vi "Teleop - shooter (SubVI).vi"(0 "Shoot":bool, 1 "inAuto":bool, 2 "AutoTurret":dbl, 7 "Desired cluster In":T1 {"shooterMotorMode" items=["PercentOutput"=0, "Position"=1, "Velocity"=2, "Current"=3, "Follower"=5, "MotionProfile"=6, "MotionMagic"=7, "MotionProfileArc"=10, "Disabled"=15]}, 9 "Constant Cluster":T4 {"12. Auton Deriv Drive Straight Gain" format="%_6f"; "11. Auton Int Drive Straight Gain" format="%_6f"; "10. Auton Prop Drive Straight Gain" format="%_6f"; "9. Auton I Output Limit Turn Gain" format="%_6f"; "8. Auton Deriv Turn Gain" format="%_6f"; "7. Auton Int Turn Gain" format="%_6f"; "1. Auton Prop Drive Gain" format="%_6f"; "2. Auton Int Drive Gain" format="%_6f"; "3. Auton Deriv Drive Gain" format="%_6f"; "4. I Output Drive  Limit" format="%_6f"; "5. Auto Drive Cheat (%)" format="%_6f"; "6. Auton Prop Turn Gain" format="%_6f"}, 11 "Sensors In":T5, 12 "wallShoot":bool, 14 "wallShootDistanceReached":bool) -> (4 "Shooting Conditions":T3, 8 "Desired cluster out":T1 {"shooterMotorMode" items=["PercentOutput"=0, "Position"=1, "Velocity"=2, "Current"=3, "Follower"=5, "MotionProfile"=6, "MotionMagic"=7, "MotionProfileArc"=10, "Disabled"=15]}, 10 "Constant Cluster Out":T4 {"12. Auton Deriv Drive Straight Gain" format="%_6f"; "11. Auton Int Drive Straight Gain" format="%_6f"; "10. Auton Prop Drive Straight Gain" format="%_6f"; "9. Auton I Output Limit Turn Gain" format="%_6f"; "8. Auton Deriv Turn Gain" format="%_6f"; "7. Auton Int Turn Gain" format="%_6f"; "1. Auton Prop Drive Gain" format="%_6f"; "2. Auton Int Drive Gain" format="%_6f"; "3. Auton Deriv Drive Gain" format="%_6f"; "4. I Output Drive  Limit" format="%_6f"; "5. Auto Drive Cheat (%)" format="%_6f"; "6. Auton Prop Turn Gain" format="%_6f"}, 15 "Sensors Out":T5)   [LabVIEW 2019]
uses:
  Autonomous/TypeDefs/Sensor TypeDef.ctl
  Disabled/Constant VI_s/Disabled - Constant Cluster Typedef.ctl
  Desired Cluster.ctl
  <vilib>/Rock Robotics/WPI/ThirdParty/Phoenix-LabVIEW/Motor Controller/Controls/CTRE_Phoenix_MotorControl_ControlMode.ctl
  <vilib>/Rock Robotics/Network Tables/NT Write Number.vi
panel:
  in  "input cluster":T3
  out "Wall Shot Shooter\nSpeed in Range":bool
  out "Wall Shot Turrent\nAngle in Range":bool
  out "Wall Shot Hood\nAngle in Range":bool
  out "Shooter Speed\nin Shooting Range":bool
  out "Turret Angle In\nShooting Range":bool
  out "Hood Angle In\nShooting Range":bool
  out "v*slope multiple":dbl
  out "x*slope multiple":dbl
  in  "v slope":dbl=0.35
  in  "x slope":dbl=-1.5
  out "desired hood angle":dbl
  out "velocity":dbl
  out "Horizontal Distance\nTo Target":dbl
  # "Inputs"
  # "Outputs"
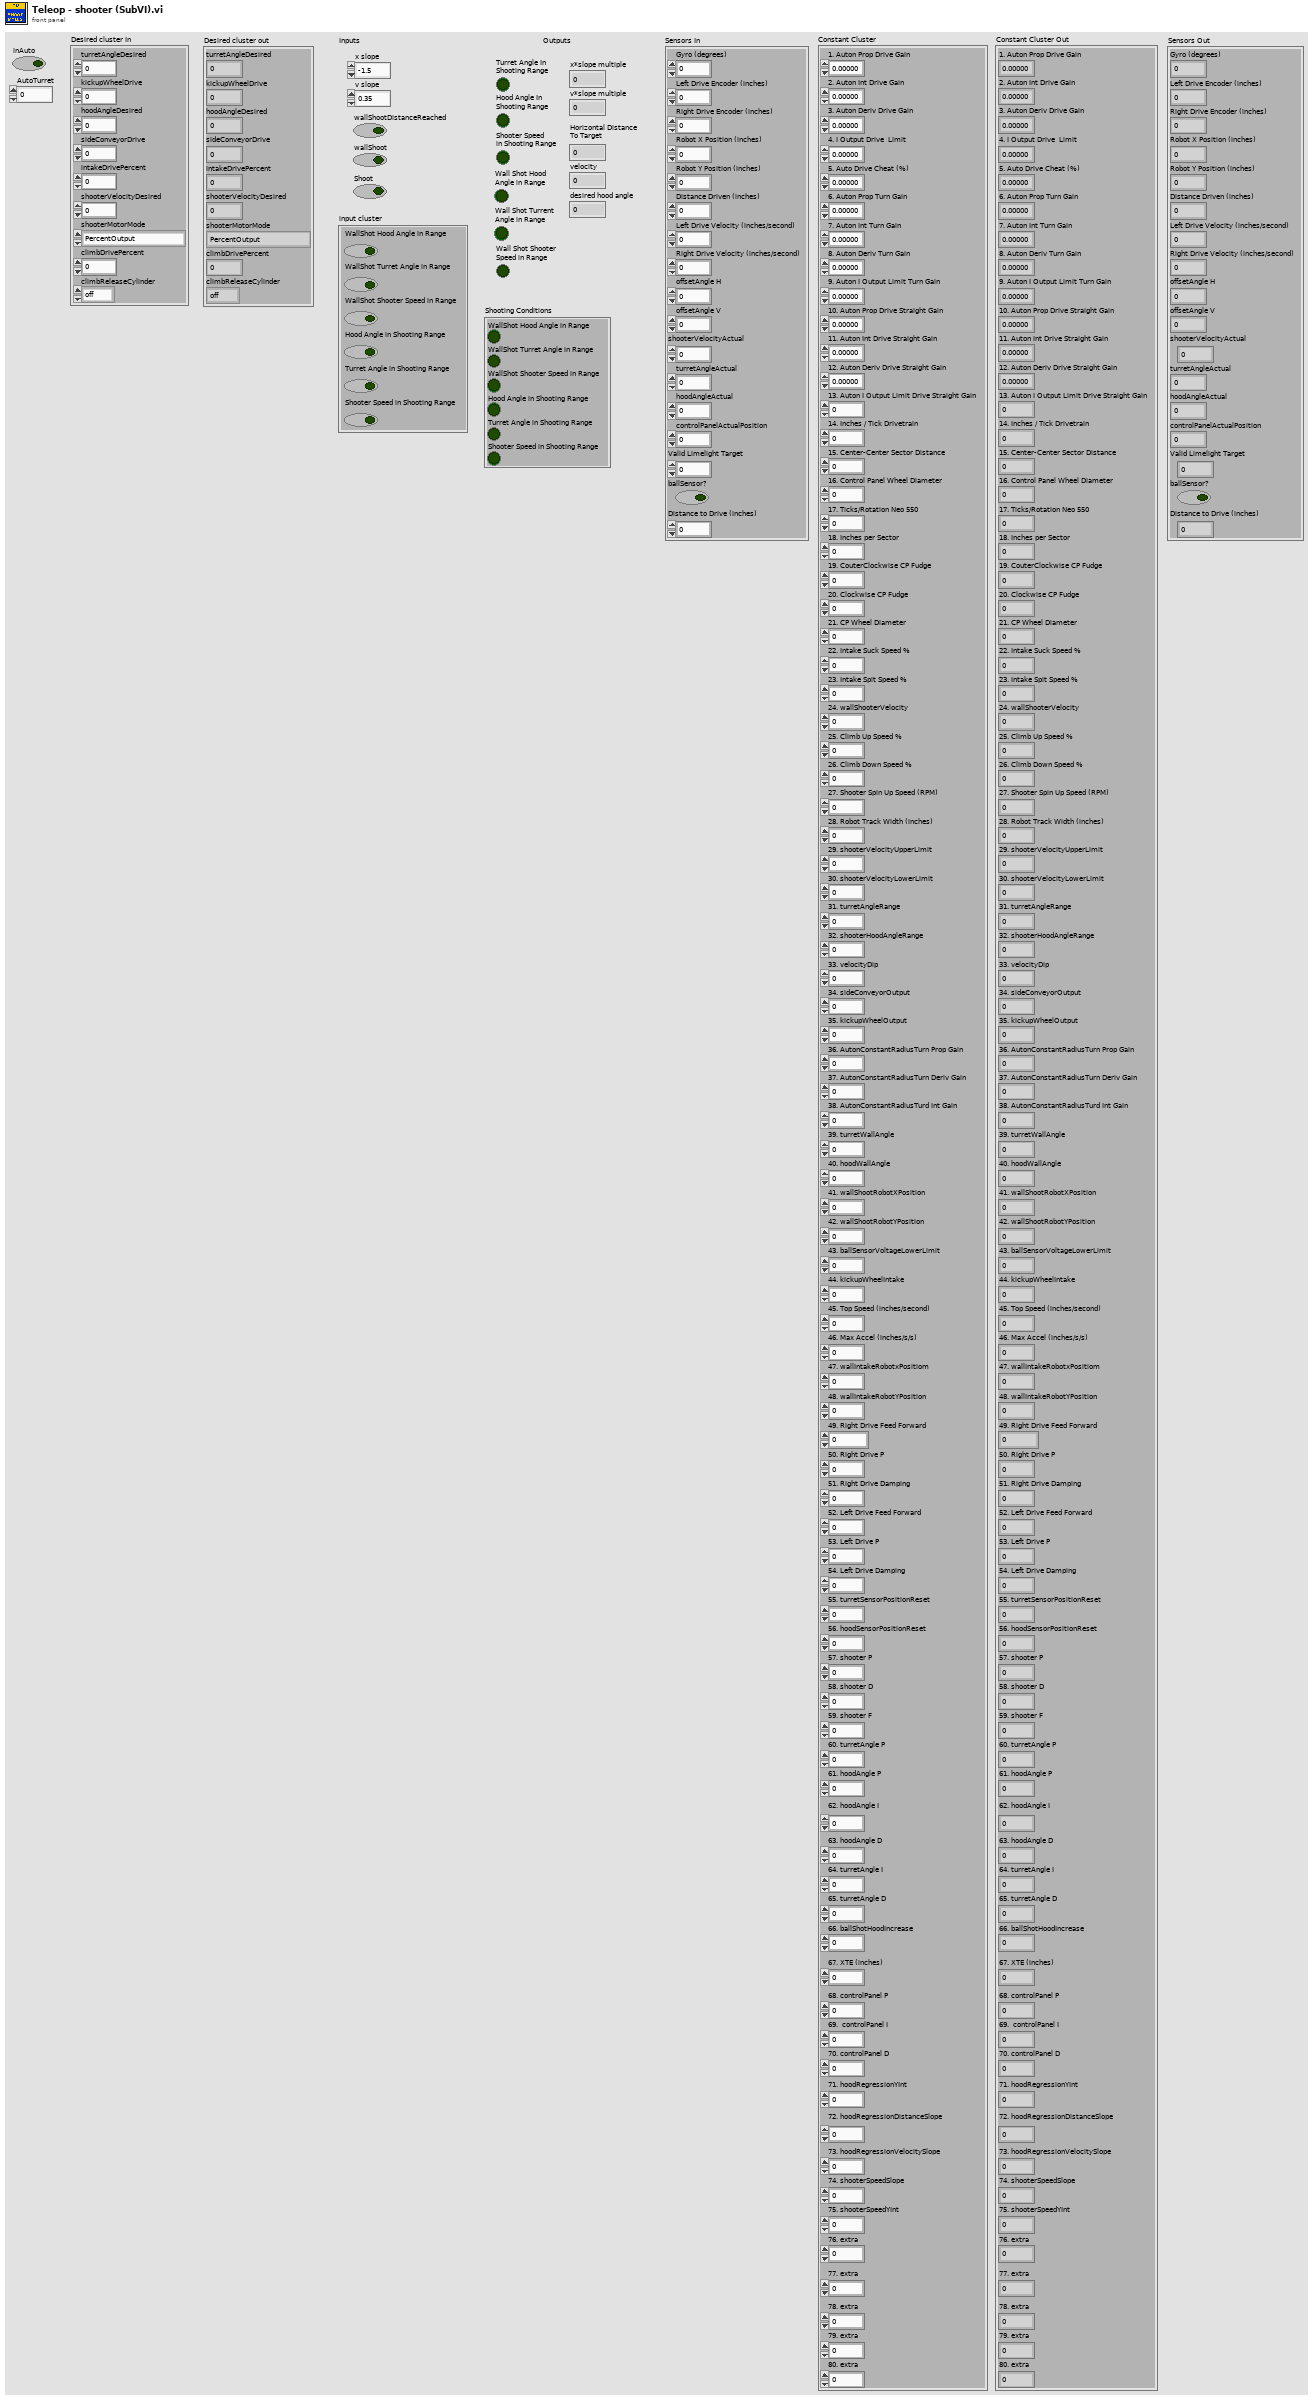
[diagram p1: front panel]
types:
  T1 = typedef "Desired Cluster.ctl" = cluster{"turretAngleDesired":dbl, "kickupWheelDrive":dbl, "hoodAngleDesired":dbl, "sideConveyorDrive":dbl, "intakeDrivePercent":dbl, "shooterVelocityDesired":dbl, "shooterMotorMode":T2, "climbDrivePercent":dbl, "climbReleaseCylinder":enum16{"off", "on", "forward", "back"}}
  T2 = typedef "CTRE_Phoenix_MotorControl_ControlMode.ctl" = u16
  T3 = cluster{"WallShot Hood Angle in Range":bool, "WallShot Turret Angle in Range":bool, "WallShot Shooter Speed in Range":bool, "Hood Angle in Shooting Range":bool, "Turret Angle in Shooting Range":bool, "Shooter Speed in Shooting Range":bool}
  T4 = typedef "Disabled - Constant Cluster Typedef.ctl" = cluster{"1. Auton Prop Drive Gain":dbl, "2. Auton Int Drive Gain":dbl, "3. Auton Deriv Drive Gain":dbl, "4. I Output Drive  Limit":dbl, "5. Auto Drive Cheat (%)":dbl, "6. Auton Prop Turn Gain":dbl, "7. Auton Int Turn Gain":dbl, "8. Auton Deriv Turn Gain":dbl, "9. Auton I Output Limit Turn Gain":dbl, "10. Auton Prop Drive Straight Gain":dbl, "11. Auton Int Drive Straight Gain":dbl, "12. Auton Deriv Drive Straight Gain":dbl, "13. Auton I Output Limit Drive Straight Gain":dbl, "14. Inches / Tick Drivetrain":dbl, "15. Center-Center Sector Distance":dbl, "16. Control Panel Wheel Diameter":dbl, "17. Ticks/Rotation Neo 550":dbl, "18. Inches per Sector":dbl, "19. CouterClockwise CP Fudge":dbl, "20. Clockwise CP Fudge":dbl, "21. CP Wheel Diameter":dbl, "22. Intake Suck Speed %":dbl, "23. Intake Spit Speed %":dbl, "24. wallShooterVelocity":dbl, "25. Climb Up Speed %":dbl, "26. Climb Down Speed %":dbl, "27. Shooter Spin Up Speed (RPM)":dbl, "28. Robot Track Width (inches)":dbl, "29. shooterVelocityUpperLimit":dbl, "30. shooterVelocityLowerLimit":dbl, "31. turretAngleRange":dbl, "32. shooterHoodAngleRange":dbl, "33. velocityDip":dbl, "34. sideConveyorOutput":dbl, "35. kickupWheelOutput":dbl, "36. AutonConstantRadiusTurn Prop Gain":dbl, "37. AutonConstantRadiusTurn Deriv Gain":dbl, "38. AutonConstantRadiusTurd Int Gain":dbl, "39. turretWallAngle":dbl, "40. hoodWallAngle":dbl, "41. wallShootRobotXPosition":dbl, "42. wallShootRobotYPosition":dbl, "43. ballSensorVoltageLowerLimit":dbl, "44. kickupWheelIntake":dbl, "45. Top Speed (inches/second)":dbl, "46. Max Accel (inches/s/s)":dbl, "47. wallIntakeRobotxPositiom":dbl, "48. wallIntakeRobotYPosition":dbl, "49. Right Drive Feed Forward":dbl, "50. Right Drive P":dbl, "51. Right Drive Damping":dbl, "52. Left Drive Feed Forward":dbl, "53. Left Drive P":dbl, "54. Left Drive Damping":dbl, "55. turretSensorPositionReset":dbl, "56. hoodSensorPositionReset":dbl, "57. shooter P":dbl, "58. shooter D":dbl, "59. shooter F":dbl, "60. turretAngle P":dbl, "61. hoodAngle P":dbl, "62. hoodAngle I":dbl, "63. hoodAngle D":dbl, "64. turretAngle I":dbl, "65. turretAngle D":dbl, "66. ballShotHoodIncrease":dbl, "67. XTE (inches)":dbl, "68. controlPanel P":dbl, "69.  controlPanel I":dbl, "70. controlPanel D":dbl, "71. hoodRegressionYInt":dbl, "72. hoodRegressionDistanceSlope":dbl, "73. hoodRegressionVelocitySlope":dbl, "74. shooterSpeedSlope":dbl, "75. shooterSpeedYInt":dbl, "76. extra":dbl, "77. extra":dbl, "78. extra":dbl, "79. extra":dbl, "80. extra":dbl}
  T5 = typedef "Sensor TypeDef.ctl" = cluster{"Gyro (degrees)":dbl, "Left Drive Encoder (inches)":dbl, "Right Drive Encoder (inches)":dbl, "Robot X Position (inches)":dbl, "Robot Y Position (inches)":dbl, "Distance Driven (inches)":dbl, "Left Drive Velocity (inches/second)":dbl, "Right Drive Velocity (inches/second)":dbl, "offsetAngle H":dbl, "offsetAngle V":dbl, "shooterVelocityActual":dbl, "turretAngleActual":dbl, "hoodAngleActual":dbl, "controlPanelActualPosition":dbl, "Valid Limelight Target":dbl, "ballSensor?":bool, "Distance to Drive (inches)":dbl}
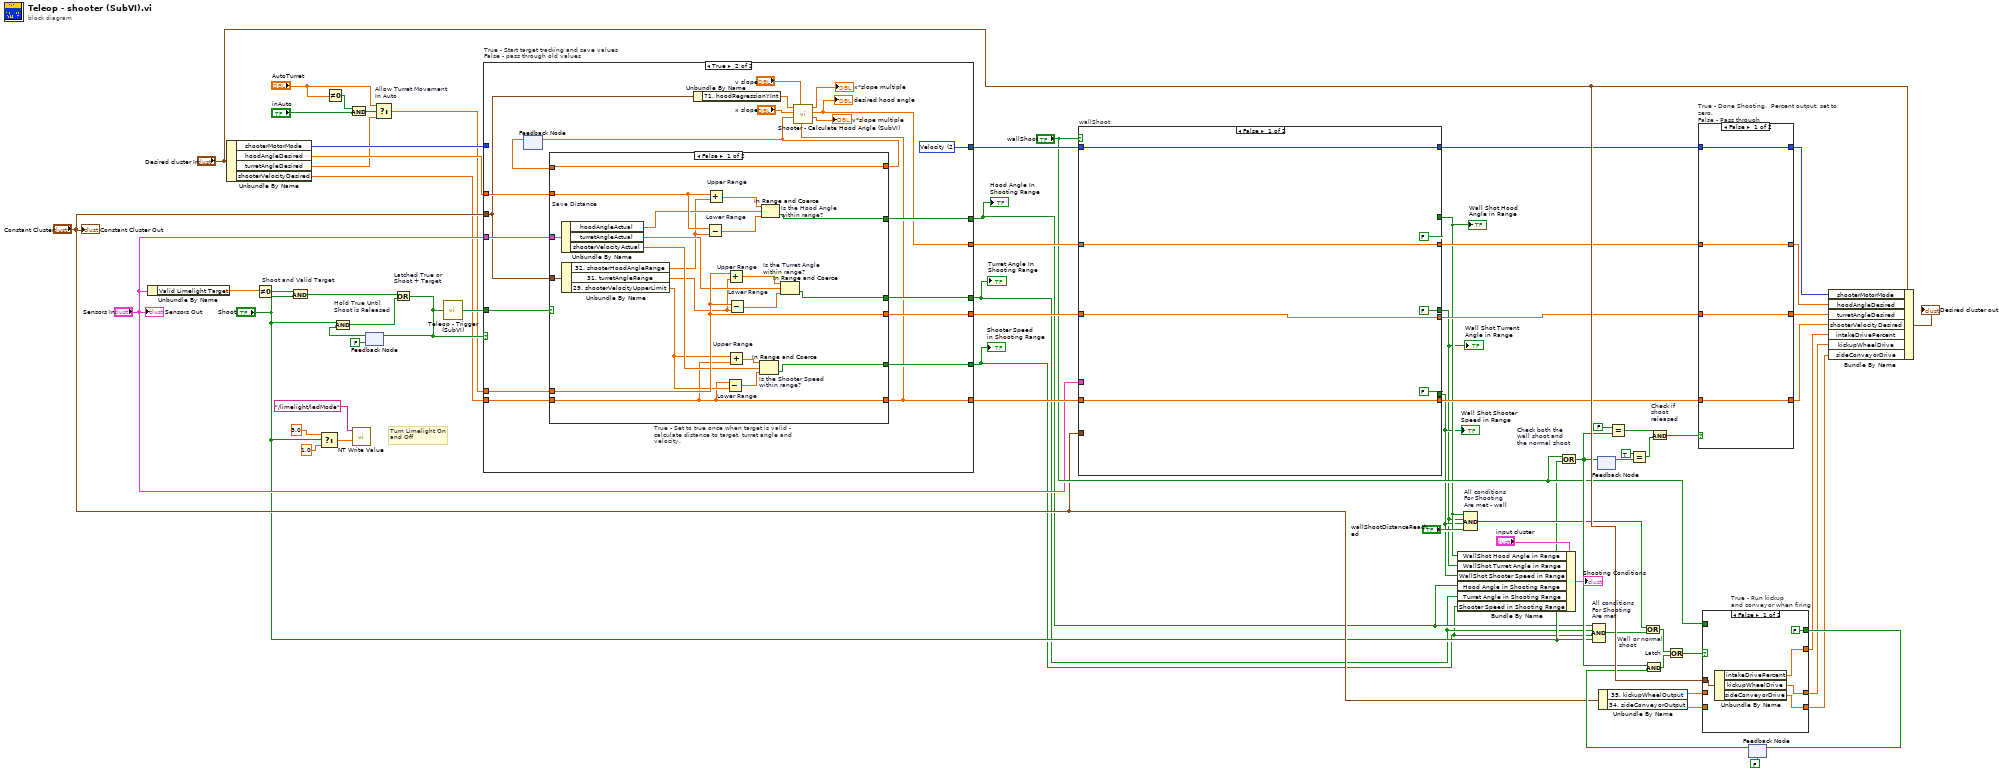
[diagram p0: block diagram]
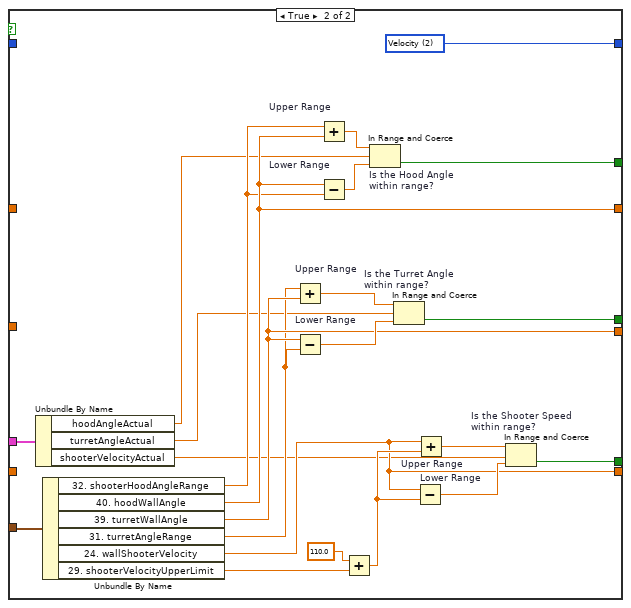
[diagram p2: hidden frame]
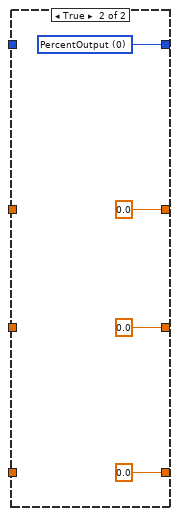
[diagram p3: hidden frame]
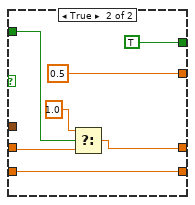
[diagram p4: hidden frame]
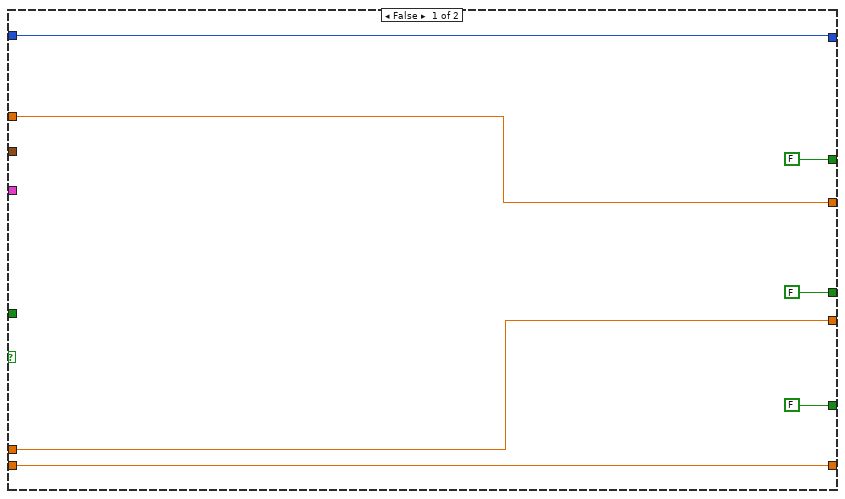
[diagram p5: hidden frame]
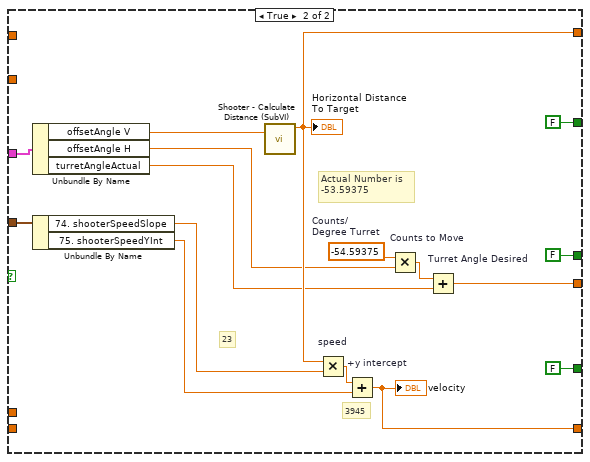
[diagram p6: hidden frame]
diagram:
  # "Turn Limelight On\nand Off"
  n1 = Unbundle By Name("Sensors In") -> ("Valid Limelight Target"=w35:dbl)
  n2 = Unbundle By Name("Desired cluster In") -> ("shooterMotorMode"=w20:T2, "hoodAngleDesired"=w19:dbl, "turretAngleDesired"=w7:dbl, "shooterVelocityDesired"=w18:dbl)
  n3 = Not Equal To 0?(x=w35) -> (x != 0?=w65:bool)
  n4 = And "Shoot and Valid Target"(x=w65, y="Shoot") -> (x .and. y?=w34:bool)
  n5 = Select(t=3.0 ("Numeric"), s="Shoot", f=1.0 ("Numeric")) -> (s? t:f=w58:dbl)
  n6 = Not Equal To 0?(x="AutoTurret") -> (x != 0?=w8:bool)
  n7 = And(x=w8, y="inAuto") -> (x .and. y?=w9:bool)
  n8 = call-poly <vilib>:"NT Write Value.vi"("Numeric"=w58, "Name"="/limelight/ledMode") -> ()  [unwired: 9 in, 1 out]
  n9 = feedback #1(FALSE) -> (w32:bool)
  n10 = And "Hold True Until\nShoot is Released"(x="Shoot", y=w32) -> (x .and. y?=w33:bool)
  n11 = Select "Allow Turret Movement\nIn Auto"(t="AutoTurret", s=w9, f=w7) -> (s? t:f=w6:dbl)
  n12 = Or "Latched True or\nShoot + Target"(x=w34, y=w33) -> (x .or. y?=w40:bool)
  n13 = feedback-in #1(w40) -> ()
  n14 = call "Teleop - Trigger (SubVI).vi"("Trigger"=w40) -> ("Trigger Output"=w67:bool)
  n15 = case "True - Start target tracking and save values\nFalse - pass through old values" shown="True" w40 {
    tunnel: [w71 w95] -> w48
    tunnel: [w69 w88] -> w50
    tunnel: w6 -> [w71 w94]
    tunnel: w19 -> [w69 w93]
    tunnel: w67 -> [_ w84]
    tunnel: w18 -> [w75 w92]
    tunnel: [w75 w76] -> w46
    tunnel: [FALSE w91] -> w3
    tunnel: [FALSE w90] -> w2
    tunnel: [FALSE w89] -> w1
    tunnel: [w70 w87] -> w44
    tunnel: w20 -> [w70 _]
    tunnel: "Sensors In" -> [_ w81]
    tunnel: "Constant Cluster" -> [_ w79]
    frame False {
    }
    frame True {
      w87 = T2 2 items=["PercentOutput"=0, "Position"=1, "Velocity"=2, "Current"=3, "Follower"=5, "MotionProfile"=6, "MotionMagic"=7, "MotionProfileArc"=10, "Disabled"=15] ("shooterMotorModeInput")
      n16 = feedback #2 "Save Distance"() -> (w85:dbl)  [unwired: 1 in]
      n17 = case "True - Set to true once when target is valid - calculate distance to target, turret angle and velocity." shown="False" w84 {
        tunnel: [w114 w126] -> w95
        tunnel: w94 -> [w114 _]
        tunnel: w93 -> [w108 _]
        tunnel: w92 -> [w97 _]
        tunnel: [w97 w125] -> w76
        tunnel: [w112 FALSE] -> w91
        tunnel: [w111 FALSE] -> w90
        tunnel: [w110 FALSE] -> w89
        tunnel: [w107 w124] -> w86
        tunnel: w85 -> [w107 _]
        tunnel: w81 -> [w105 w120]
        tunnel: w79 -> [w101 w123]
        frame False {
          n18 = Unbundle By Name(w105) -> ("hoodAngleActual"=w104:dbl, "turretAngleActual"=w103:dbl, "shooterVelocityActual"=w102:dbl)
          n19 = Unbundle By Name(w101) -> ("32. shooterHoodAngleRange"=w100:dbl, "31. turretAngleRange"=w99:dbl, "29. shooterVelocityUpperLimit"=w98:dbl)
          n20 = Subtract "Lower Range"(x=w108, y=w100) -> (x-y=w113:dbl)
          n21 = Add "Upper Range"(x=w108, y=w100) -> (x+y=w106:dbl)
          n22 = Subtract "Lower Range"(x=w97, y=w98) -> (x-y=w96:dbl)
          n23 = Add "Upper Range"(x=w114, y=w99) -> (x+y=w115:dbl)
          n24 = Add "Upper Range"(x=w98, y=w97) -> (x+y=w109:dbl)
          n25 = Subtract "Lower Range"(x=w114, y=w99) -> (x-y=w116:dbl)
          n26 = In Range and Coerce "Is the Shooter Speed\nwithin range?"(upper limit=w109, x=w102, lower limit=w96) -> (In Range?=w110:bool)  [unwired: 1 out]
          n27 = In Range and Coerce "Is the Hood Angle\nwithin range?"(upper limit=w106, x=w104, lower limit=w113) -> (In Range?=w112:bool)  [unwired: 1 out]
          n28 = In Range and Coerce "Is the Turret Angle\nwithin range?"(upper limit=w115, x=w103, lower limit=w116) -> (In Range?=w111:bool)  [unwired: 1 out]
        }
        frame True {
          w131 = -54.59375  # Counts/ Degree Turret
          # "23"
          # "3945"
          # "Actual Number is\n-53.59375"
          n29 = Unbundle By Name(w120) -> ("offsetAngle V"=w118:dbl, "offsetAngle H"=w119:dbl, "turretAngleActual"=w117:dbl)
          n30 = Unbundle By Name(w123) -> ("74. shooterSpeedSlope"=w121:dbl, "75. shooterSpeedYInt"=w122:dbl)
          n31 = call "Shooter - Calculate Distance (SubVI).vi"("offsetAngle V"=w118) -> ("Distance (inches)"=w124:dbl)  [unwired: 10 in]
          "Horizontal Distance\nTo Target" <- w124
          n32 = Multiply "speed"(x=w124, y=w121) -> (x*y=w130:dbl)
          n33 = Add "+y intercept"(x=w130, y=w122) -> (x+y=w125:dbl)
          "velocity" <- w125
          n34 = Multiply "Counts to Move"(x=w131, y=w119) -> (x*y=w132:dbl)
          n35 = Add "Turret Angle Desired"(x=w132, y=w117) -> (x+y=w126:dbl)
        }
      }
      n36 = feedback-in #2(w86) -> ()
      n37 = Unbundle By Name(w79) -> ("71. hoodRegressionYInt"=w80:dbl)
      n38 = call "Shooter - Calculate Hood Angle (SubVI).vi"("shooterVelocityDesired In"=w76, "v slope"="v slope", "distance in"=w86, "x slope"="x slope", "71. hoodRegressionYInt"=w80) -> ("v*slope multiple"=→"v*slope multiple":dbl, "hood counts"=w88:dbl, "x*slope multiple"=→"x*slope multiple":dbl)  [unwired: 4 in]
      "desired hood angle" <- w88
    }
  }
  "Hood Angle In\nShooting Range" <- w3
  "Turret Angle In\nShooting Range" <- w2
  "Shooter Speed\nin Shooting Range" <- w1
  n39 = case "wallShoot" shown="False" "wallShoot" {
    tunnel: w50 -> [w138 _]
    tunnel: [w138 w152] -> w49
    tunnel: w48 -> [w137 _]
    tunnel: [w137 w151] -> w47
    tunnel: w46 -> [w136 _]
    tunnel: [w136 w146] -> w45
    tunnel: w44 -> [w139 _]
    tunnel: [w139 w162] -> w43
    tunnel: "Constant Cluster" -> [_ w161]
    tunnel: [FALSE w155] -> w25
    tunnel: [FALSE w154] -> w26
    tunnel: [FALSE w153] -> w24
    tunnel: "Sensors In" -> [_ w143]
    frame False {
    }
    frame True {
      w162 = T2 2 items=["PercentOutput"=0, "Position"=1, "Velocity"=2, "Current"=3, "Follower"=5, "MotionProfile"=6, "MotionMagic"=7, "MotionProfileArc"=10, "Disabled"=15] ("shooterMotorModeInput")
      n40 = Unbundle By Name(w143) -> ("hoodAngleActual"=w142:dbl, "turretAngleActual"=w141:dbl, "shooterVelocityActual"=w140:dbl)
      n41 = Unbundle By Name(w161) -> ("32. shooterHoodAngleRange"=w147:dbl, "40. hoodWallAngle"=w152:dbl, "39. turretWallAngle"=w151:dbl, "31. turretAngleRange"=w145:dbl, "24. wallShooterVelocity"=w146:dbl, "29. shooterVelocityUpperLimit"=w144:dbl)
      n42 = Add "Upper Range"(x=w145, y=w151) -> (x+y=w159:dbl)
      n43 = Subtract "Lower Range"(x=w151, y=w145) -> (x-y=w160:dbl)
      n44 = Add "Upper Range"(x=w147, y=w152) -> (x+y=w157:dbl)
      n45 = Subtract "Lower Range"(x=w152, y=w147) -> (x-y=w158:dbl)
      n46 = Add(x=110.0, y=w144) -> (x+y=w148:dbl)
      n47 = In Range and Coerce "Is the Hood Angle\nwithin range?"(upper limit=w157, x=w142, lower limit=w158) -> (In Range?=w154:bool)  [unwired: 1 out]
      n48 = In Range and Coerce "Is the Turret Angle\nwithin range?"(upper limit=w159, x=w141, lower limit=w160) -> (In Range?=w153:bool)  [unwired: 1 out]
      n49 = Subtract "Lower Range"(x=w146, y=w148) -> (x-y=w156:dbl)
      n50 = Add "Upper Range"(x=w146, y=w148) -> (x+y=w149:dbl)
      n51 = In Range and Coerce "Is the Shooter Speed\nwithin range?"(upper limit=w149, x=w140, lower limit=w156) -> (In Range?=w155:bool)  [unwired: 1 out]
    }
  }
  "Wall Shot Hood\nAngle in Range" <- w26
  "Wall Shot Turrent\nAngle in Range" <- w24
  "Wall Shot Shooter\nSpeed in Range" <- w25
  n52 = Bundle By Name(cluster="input cluster", "WallShot Hood Angle in Range"=w26, "WallShot Turret Angle in Range"=w24, "WallShot Shooter Speed in Range"=w25, "Hood Angle in Shooting Range"=w3, "Turret Angle in Shooting Range"=w2, "Shooter Speed in Shooting Range"=w1) -> (→"Shooting Conditions":T3)
  n53 = Compound Arithmetic op=AND "All conditions\nFor Shooting\nAre met - wall"(w26, w24, w25, "wallShootDistanceReached") -> (w28:bool)
  n54 = Or "Check both the \nwall shoot and \nthe normal shoot"(x="wallShoot", y="Shoot") -> (x .or. y?=w38:bool)
  n55 = Compound Arithmetic op=AND "All conditions\nFor Shooting\nAre met"(w3, w2, w1, "Shoot") -> (w29:bool)
  n56 = feedback-in #3(w38) -> ()
  n57 = feedback #3() -> (w55:bool)  [unwired: 1 in]
  n58 = Unbundle By Name("Constant Cluster") -> ("35. kickupWheelOutput"=w30:dbl, "34. sideConveyorOutput"=w66:dbl)
  n59 = Equal?(x=FALSE, y=w38) -> (x = y?=w53:bool)
  n60 = Equal?(x=TRUE, y=w55) -> (x = y?=w52:bool)
  n61 = Or "Wall or normal\n shoot"(x=w28, y=w29) -> (x .or. y?=w41:bool)
  n62 = And "Check if \nshoot \nreleased"(x=w53, y=w52) -> (x .and. y?=w51:bool)
  n63 = case "True - Done Shooting.  Percent output, set to zero.\nFalse - Pass through" shown="False" w51 {
    tunnel: w47 -> [w165 _]
    tunnel: w49 -> [w166 _]
    tunnel: [w166 0.0 ("hoodAngleActual")] -> w15
    tunnel: [w165 0.0 ("turretAngleDesiredIn")] -> w14
    tunnel: [w164 0.0 ("shooterVelocityDesired In")] -> w13
    tunnel: w45 -> [w164 _]
    tunnel: [w163 w167] -> w16
    tunnel: w43 -> [w163 _]
    frame False {
    }
    frame True {
      w167 = T2 0 items=["PercentOutput"=0, "Position"=1, "Velocity"=2, "Current"=3, "Follower"=5, "MotionProfile"=6, "MotionMagic"=7, "MotionProfileArc"=10, "Disabled"=15] ("shooterMotorModeInput")
    }
  }
  n64 = feedback #4(FALSE) -> (w63:bool)
  n65 = And "Latch"(x=w38, y=w63) -> (x .and. y?=w64:bool)
  n66 = Or(x=w41, y=w64) -> (x .or. y?=w42:bool)
  n67 = case "True - Run kickup\nand conveyor when firing" shown="False" w42 {
    tunnel: [w172 w179] -> w11
    tunnel: [w173 w182] -> w10
    tunnel: w30 -> [_ w178]
    tunnel: w66 -> [_ w182]
    tunnel: [w171 0.5 ("Intake Motor Output")] -> w12
    tunnel: [FALSE TRUE] -> w62
    tunnel: "wallShoot" -> [_ w176]
    tunnel: "Desired cluster In" -> [w174 _]
    frame False {
      n68 = Unbundle By Name(w174) -> ("intakeDrivePercent"=w171:dbl, "kickupWheelDrive"=w172:dbl, "sideConveyorDrive"=w173:dbl)
    }
    frame True {
      n69 = Select(t=1.0, s=w176, f=w178) -> (s? t:f=w179:dbl)
    }
  }
  n70 = feedback-in #4(w62) -> ()
  n71 = Bundle By Name(cluster="Desired cluster In", "shooterMotorMode"=w16, "hoodAngleDesired"=w15, "turretAngleDesired"=w14, "shooterVelocityDesired"=w13, "intakeDrivePercent"=w12, "kickupWheelDrive"=w11, "sideConveyorDrive"=w10) -> (→"Desired cluster out":T1)
  "Sensors Out" <- "Sensors In"
  "Constant Cluster Out" <- "Constant Cluster"
